vi "向excel报表填数据.vi"(6 "报告抬头":string, 8 "错误输入（无错误）":errorcluster caption="error out", 9 "报表路径":path, 10 "Cluster引用句柄":refnum<vi>, 11 "NI_report输入":refnum<class "NI_report.lvclass">) -> (0 "错误输出":errorcluster caption="error out", 3 "NI_report输出":refnum<class "NI_report.lvclass">)   [LabVIEW 2013]
doc: "试验得到的报表以txt形式保存，把txt数据输入到excel中，以便打印"
uses:
  <vilib>/Utility/NIReport.llb/NI_report.lvclass
  <vilib>/Utility/NIReport.llb/Append Report Text (str wrap).vi
  <vilib>/Utility/config.llb/Read Key (String).vi
  <vilib>/Utility/config.llb/NI_LVConfig.lvlib
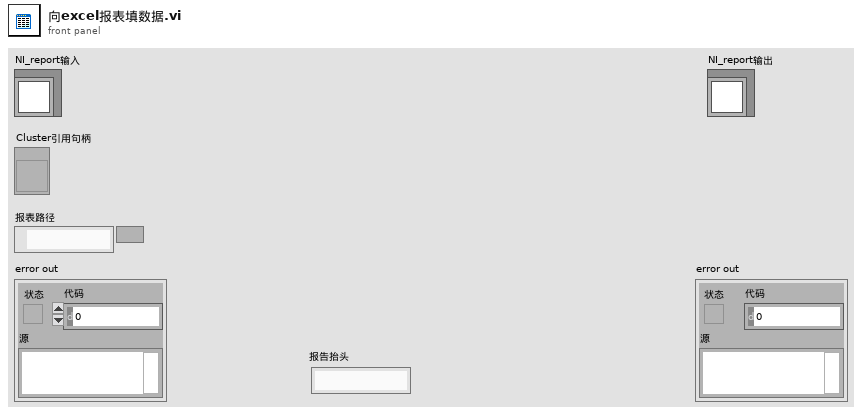
[diagram p1: front panel]
types:
  T1 = cluster{"Italic":enum16{"Italic Unchanged", "Italic On", "Italic Off"}, "Strike Through":enum16{"Strike Through Unchanged", "Strike Through On", "Strike Through Off"}, "Underline":enum16{"Underline Unchanged", "Underline On", "Underline Off"}, "Bold":enum16{"Bold Unchanged", "Bold On", "Bold Off"}}
  T2 = cluster{"Charset (-1)":i16, "Weight (-1)":i16, "Name":string, "Size":string}
  T3 = typedef "NI_LVConfig.lvlib/Config Data RefNum.ctl" = refnum<k1>
  T4 = cluster{"position (excel)":cluster{"row":i32, "column":i32}, "Label.Text":string, "bookmark (word)":string}
  T5 = cluster{"position (excel)":cluster{"row":i32, "column":i32}, "bookmark (word)":string, "bookmark (word)":string}
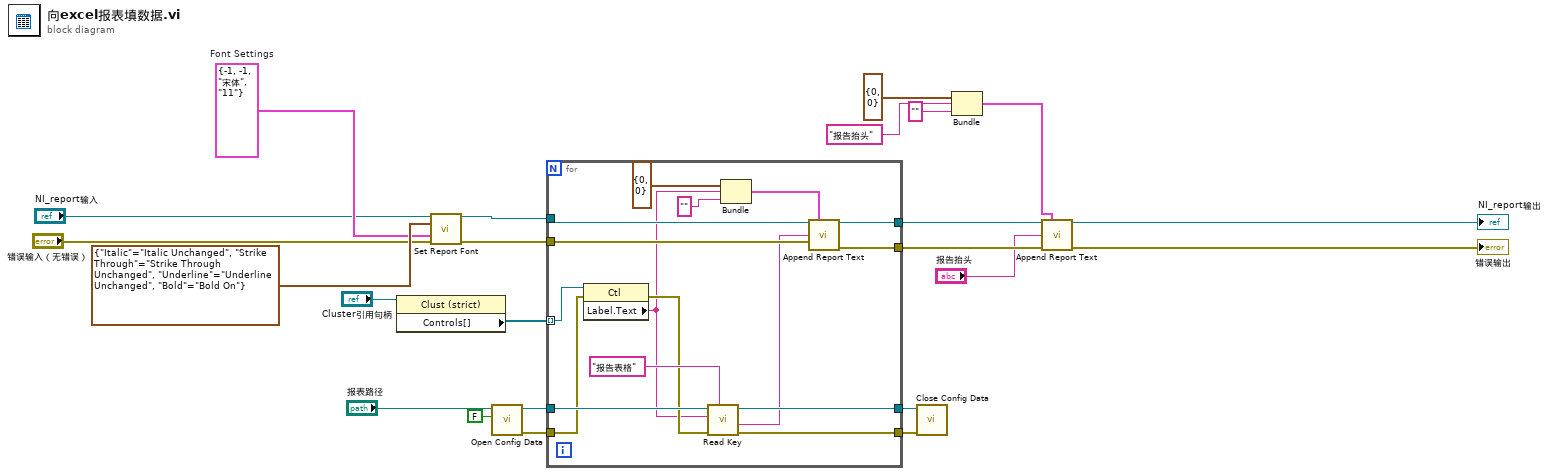
[diagram p0: block diagram]
diagram:
  w14 = T2 {"Charset (-1)"=-1, "Weight (-1)"=-1, "Name"="宋体", "Size"="11"}  # Font Settings
  n1 = property on="属性节点" class="Clust (strict)"(reference="Cluster引用句柄") -> ("Controls[]"=w19:refnum<vi>[])  [unwired: 1 in, 2 out]
  n2 = call-dynamic "Set Report Font.vi"("report in"="NI_report输入", "text options"=T1 {"Italic"=enum."Italic Unchanged", "Strike Through"=enum."Strike Through Unchanged", "Underline"=enum."Underline Unchanged", "Bold"=enum."Bold On"}, "font settings"=w14, "error in (no error)"="错误输入（无错误）") -> ("report out"=w13:refnum<class "NI_report.lvclass">, "error out"=w12:errorcluster)  [unwired: 9 in, 1 out]
  n3 = call <vilib>:"Open Config Data.vi"("create file if necessary (T)"=FALSE, "configuration file path"="报表路径") -> ("error out"=w21:errorcluster, "refnum"=w20:T3)  [unwired: 7 in, 1 out]
  n4 = for {
    tunnel: w19 -> [w39] mode=indexing
    tunnel: w20 -> [w36]
    tunnel: [w38] -> w23
    tunnel: w21 -> [w35]
    tunnel: [w33] -> w22
    tunnel: w13 -> [w32]
    tunnel: w12 -> [w31]
    tunnel: [w25] -> w9
    tunnel: [w24] -> w8
    n5 = property class="Ctl"(reference=w39, error in=w35) -> (error out=w34:errorcluster, "Label.Text"=w28:string)  [unwired: 1 out]
    n6 = call-poly <vilib>:"Read Key.vi"("section"="报告表格", "error in (no error)"=w34, "key"=w28, "refnum"=w36) -> ("error out"=w33:errorcluster, "value"=w30:string, "refnum out"=w38:T3)  [unwired: 4 in, 1 out]
    n7 = Bundle("position (excel)"=cluster{"row":i32, "column":i32} {"row"=0, "column"=0}, "Label.Text"=w28, "bookmark (word)"="") -> (w26:T4)  [unwired: 1 in]
    n8 = call-poly <vilib>:"Append Report Text.vi"("report in"=w32, "MS Office parameters"=w26, "text"=w30, "error in (no error)"=w31) -> ("report out"=w25:refnum<class "NI_report.lvclass">, "error out"=w24:errorcluster)  [unwired: 8 in, 2 out]
  }
  n9 = call <vilib>:"Close Config Data.vi"("error in (no error)"=w22, "refnum"=w23) -> ()  [unwired: 8 in, 2 out]
  n10 = Bundle("position (excel)"=cluster{"row":i32, "column":i32} {"row"=0, "column"=0}, "bookmark (word)"="报告抬头", "bookmark (word)"="") -> (w4:T5)  [unwired: 1 in]
  n11 = call-poly <vilib>:"Append Report Text.vi"("report in"=w9, "MS Office parameters"=w4, "text"="报告抬头", "error in (no error)"=w8) -> ("report out"=→"NI_report输出":refnum<class "NI_report.lvclass">, "error out"=→"错误输出":errorcluster)  [unwired: 8 in, 2 out]
